vi "Read Shift from File.vi"(8 "error in (no error)":errorcluster, 10 "XML File Path":path, 11 "Shift in":refnum<class "Shift.lvclass">) -> (0 "error out":errorcluster, 3 "Shift out":refnum<class "Shift.lvclass">)   [LabVIEW 2013]
uses:
  Shift.lvclass
  <vilib>/Utility/xml.llb/Read From XML File(string).vi
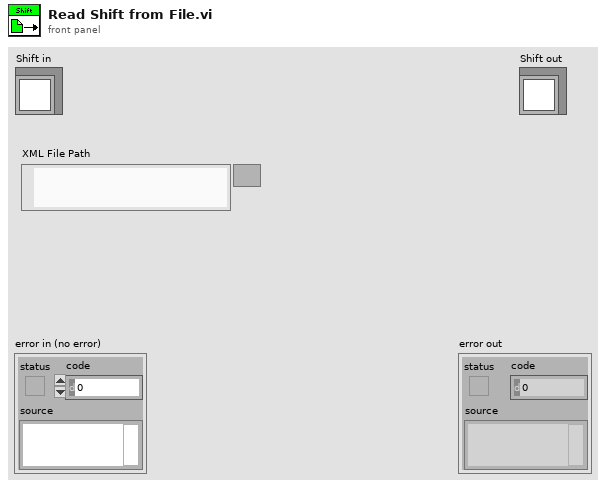
[diagram p1: front panel]
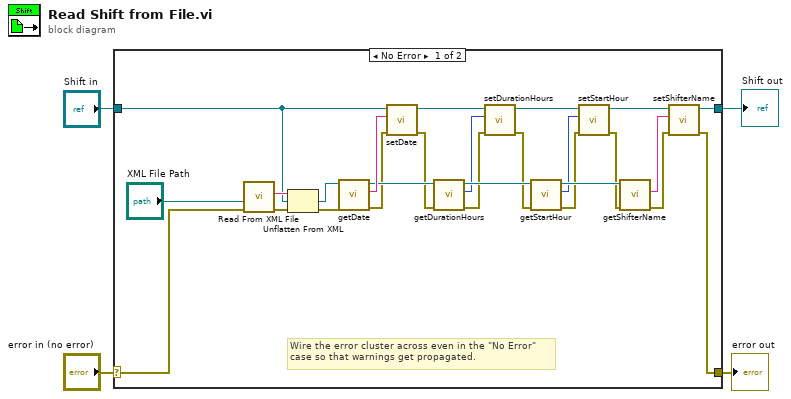
[diagram p0: block diagram]
diagram:
  n1 = case shown="No Error" "error in (no error)" {
    selector: "error in (no error)" -> [w29 w32]
    tunnel: [w5 w32] -> w3
    tunnel: [w14 w31] -> w1
    tunnel: "Shift in" -> [w23 w31]
    frame No Error {
      # "Wire the error cluster across even in the \"No Error\"\ncase so that warnings get propagated."
      n2 = call-poly <vilib>:"Read From XML File.vi"("error in (no error)"=w29, "XML File Path"="XML File Path") -> ("error out"=w28:errorcluster, "XML Elements"=w27:string)  [unwired: 7 in, 1 out]
      n3 = Unflatten From XML(xml string=w27, type=w23, error in (no error)=w28) -> (value=w25:refnum<class "Shift.lvclass">, error out=w26:errorcluster)
      n4 = call-dynamic "getDate.vi"("error in (no error)"=w26, "Shift in"=w25) -> ("error out"=w19:errorcluster, "Date"=w24:string, "Shift out"=w22:refnum<class "Shift.lvclass">)  [unwired: 7 in]
      n5 = call-dynamic "setDate.vi"("error in (no error)"=w19, "Date"=w24, "Shift in"=w23) -> ("error out"=w18:errorcluster, "Shift out"=w17:refnum<class "Shift.lvclass">)  [unwired: 7 in]
      n6 = call-dynamic "getDurationHours.vi"("error in (no error)"=w18, "Shift in"=w22) -> ("error out"=w12:errorcluster, "Duration Hours"=w13:u8, "Shift out"=w21:refnum<class "Shift.lvclass">)  [unwired: 7 in]
      n7 = call-dynamic "setDurationHours.vi"("error in (no error)"=w12, "Duration Hours"=w13, "Shift in"=w17) -> ("error out"=w11:errorcluster, "Shift out"=w16:refnum<class "Shift.lvclass">)  [unwired: 7 in]
      n8 = call-dynamic "getStartHour.vi"("error in (no error)"=w11, "Shift in"=w21) -> ("error out"=w9:errorcluster, "Start Hour"=w10:u8, "Shift out"=w20:refnum<class "Shift.lvclass">)  [unwired: 7 in]
      n9 = call-dynamic "setStartHour.vi"("error in (no error)"=w9, "Start Hour"=w10, "Shift in"=w16) -> ("error out"=w8:errorcluster, "Shift out"=w15:refnum<class "Shift.lvclass">)  [unwired: 7 in]
      n10 = call-dynamic "getShifterName.vi"("error in (no error)"=w8, "Shift in"=w20) -> ("error out"=w6:errorcluster, "Shifter Name"=w7:string)  [unwired: 7 in, 1 out]
      n11 = call-dynamic "setShifterName.vi"("error in (no error)"=w6, "Shifter Name"=w7, "Shift in"=w15) -> ("error out"=w5:errorcluster, "Shift out"=w14:refnum<class "Shift.lvclass">)  [unwired: 7 in]
    }
    frame Error {
    }
  }
  "error out" <- w3
  "Shift out" <- w1
